vi "getConfigFileDefault.vi"() -> (3 "configFileDefault":path)   [LabVIEW 2018]
doc: "Get the default configuration file."
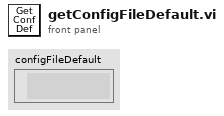
[diagram p1: front panel]
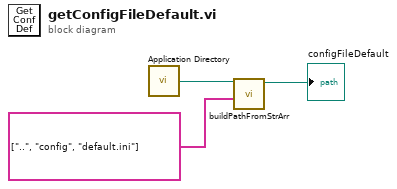
[diagram p0: block diagram]
diagram:
  n1 = call <vilib>:"Application Directory.vi"() -> ("Application Directory"=w3:path)
  n2 = call "buildPathFromStrArr.vi"("String Array"=string[] ["..", "config", "default.ini"], "Root Path"=w3) -> ("Absolute Path"=→"configFileDefault":path)  [unwired: 9 in]
